vi "Trial 4 A4 copy.vi"() -> ()   [LabVIEW 2022 SP3]
uses:
  Documents/Control 1 Trial 3.ctl
panel:
  out "Time remaining":dbl
  in  "Start":bool
  in  "Stop":bool
  in  "Washing Mode Menu":T1(ring)
  out "Washing Stage":string
  out "Washing Mode":string
  in  "On/Off":bool
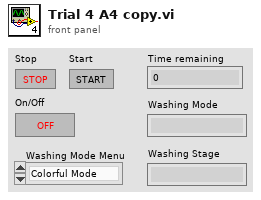
[diagram p1: front panel]
types:
  T1 = enum16{"Colorful Mode", "Intensive Mode", "Quick Wash"}
  T2 = typedef "Control 1 Trial 3.ctl" = enum16{"Off", "On", "Start Washing", "Pre-rinse", "Main Washing", "Final Spin", "Done Washing"}
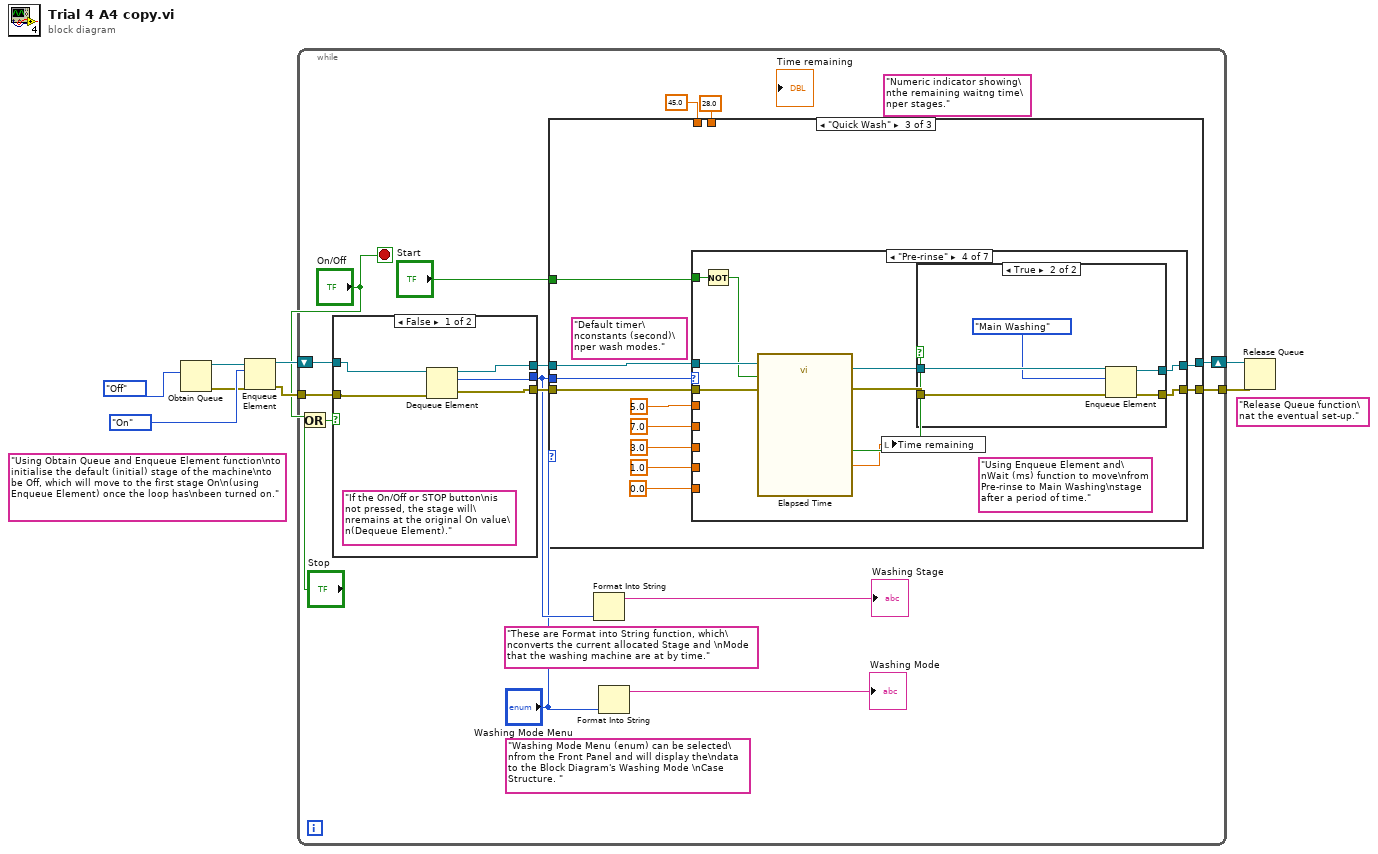
[diagram p0: block diagram]
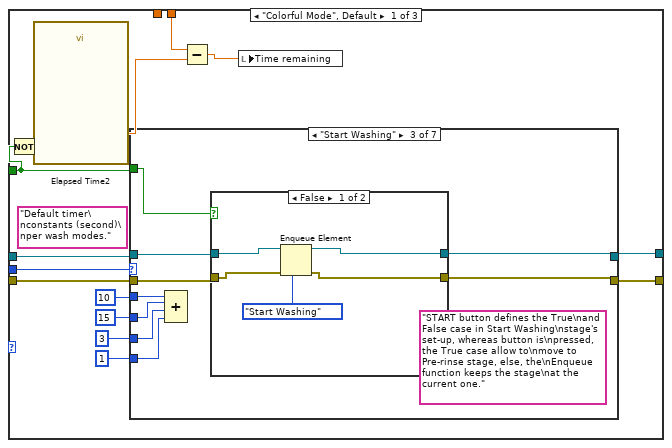
[diagram p2: hidden frame]
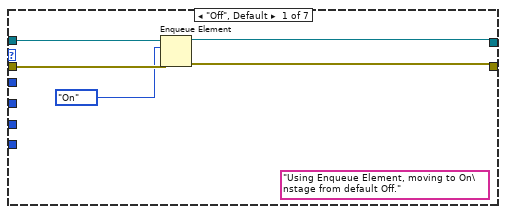
[diagram p3: hidden frame]
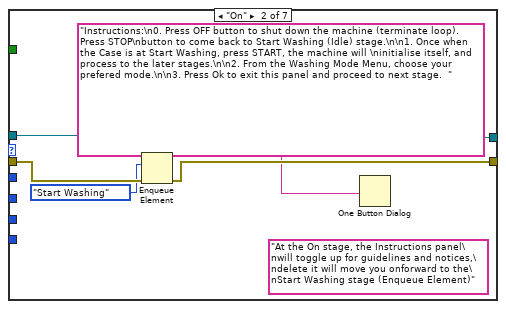
[diagram p4: hidden frame]
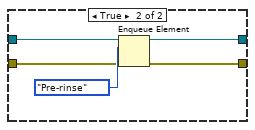
[diagram p5: hidden frame]
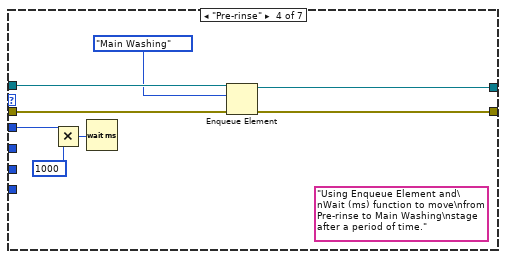
[diagram p6: hidden frame]
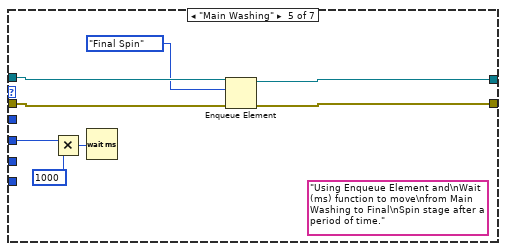
[diagram p7: hidden frame]
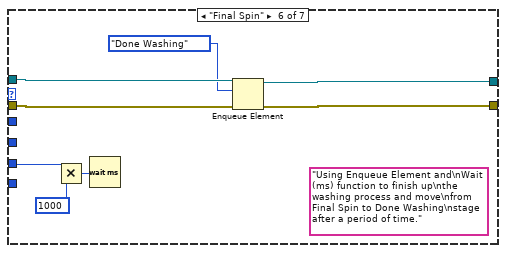
[diagram p8: hidden frame]
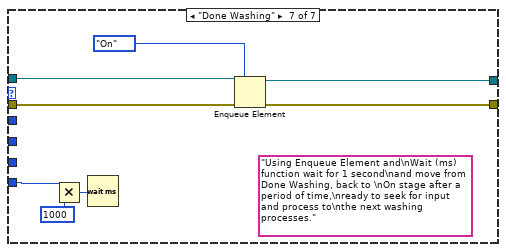
[diagram p9: hidden frame]
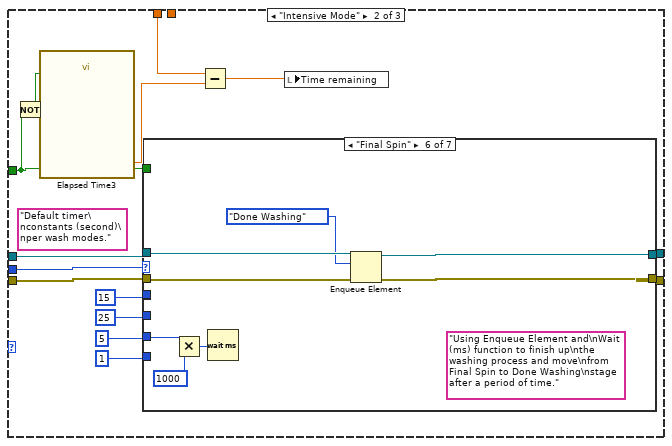
[diagram p10: hidden frame]
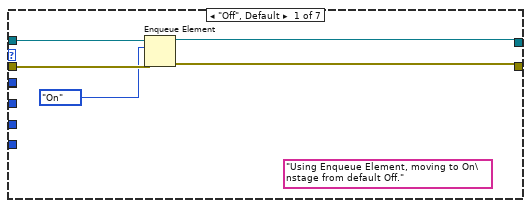
[diagram p11: hidden frame]
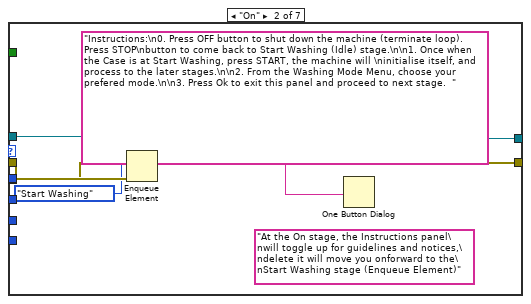
[diagram p12: hidden frame]
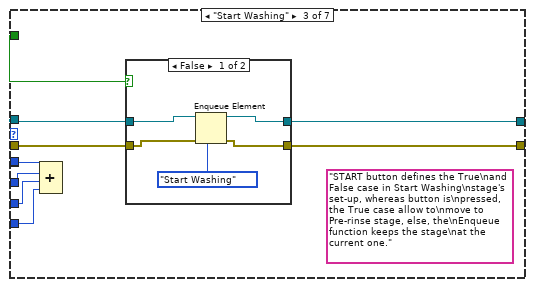
[diagram p13: hidden frame]
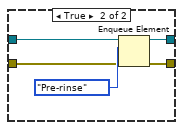
[diagram p14: hidden frame]
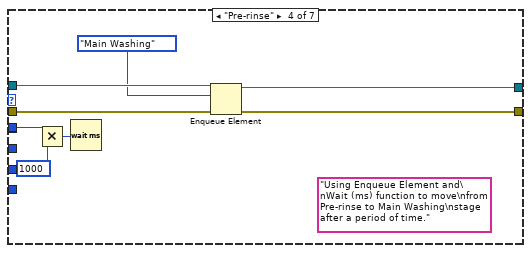
[diagram p15: hidden frame]
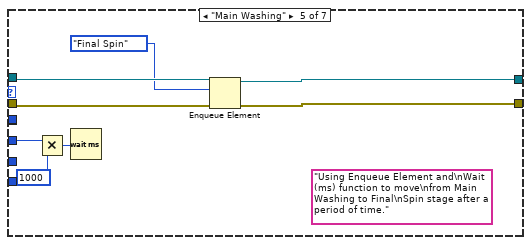
[diagram p16: hidden frame]
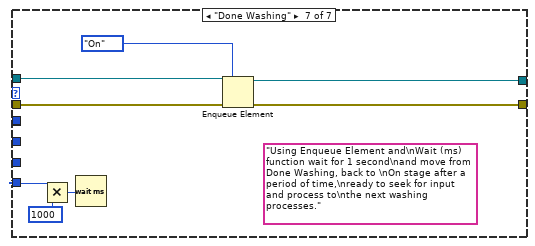
[diagram p17: hidden frame]
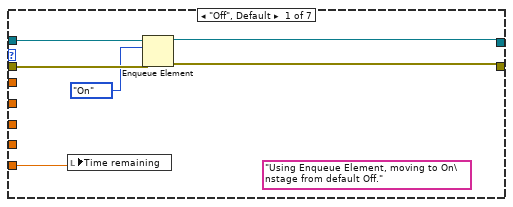
[diagram p18: hidden frame]
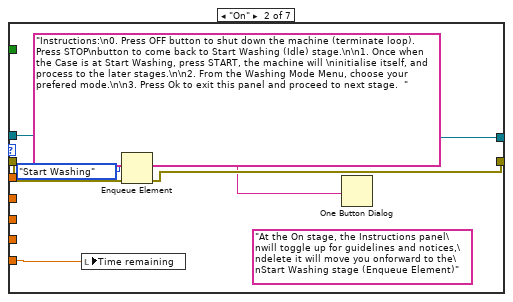
[diagram p19: hidden frame]
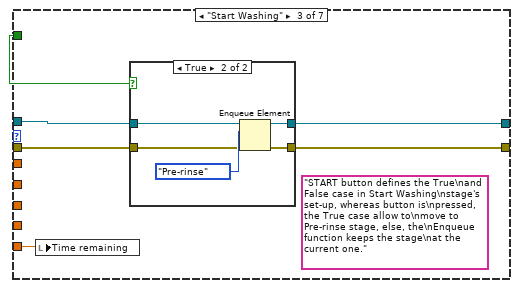
[diagram p20: hidden frame]
diagram:
  (unwired) "Release Queue function\nat the eventual set-up."
  (unwired) "Using Obtain Queue and Enqueue Element function\nto initialise the default (initial) stage of the machine\nto be Off, which will move to the first stage On\n(using Enqueue Element) once the loop has\nbeen turned on."
  n1 = Obtain Queue(element data type=Control_1_Trial_3."Off") -> (queue out=w8:refnum<queue>, error out=w2:errorcluster)  [unwired: 4 in, 1 out]
  n2 = Enqueue Element(queue=w8, element=Control_1_Trial_3."On", error in (no error)=w2) -> (queue out=w7:refnum<queue>, error out=w1:errorcluster)  [unwired: 1 in, 1 out]
  n3 = while {
    shift-right: [w18] -> w5
    shift-left: w7 -> [w23]
    tunnel: w1 -> [w24]
    tunnel: [w17] -> w6
    stop <- "On/Off" stop-if-true
    (unwired) "Numeric indicator showing\nthe remaining waitng time\nper stages."
    (unwired) "Washing Mode Menu (enum) can be selected\nfrom the Front Panel and will display the\ndata to the Block Diagram's Washing Mode \nCase Structure. "
    (unwired) "These are Format into String function, which\nconverts the current allocated Stage and \nMode that the washing machine are at by time."
    n4 = Or(x="On/Off", y="Stop") -> (x .or. y?=w16:bool)
    n5 = case shown="False" w16 {
      tunnel: w24 -> [w291 w296]
      tunnel: w23 -> [w292 w297]
      tunnel: [w288 w294] -> w21
      tunnel: [w289 w295] -> w20
      tunnel: [w290 Control_1_Trial_3."Off"] -> w15
      frame False {
        (unwired) "If the On/Off or STOP button\nis not pressed, the stage will\nremains at the original On value\n(Dequeue Element)."
        n6 = Dequeue Element(queue=w292, error in (no error)=w291) -> (queue out=w288:refnum<queue>, element=w290:T2, error out=w289:errorcluster)  [unwired: 1 in, 1 out]
      }
      frame True {
        (unwired) "Else if the On/Off or STOP button\nis  pressed, the stage will then\nmove to Off value (Flush Queue)."
        n7 = Flush Queue(queue=w297, error in (no error)=w296) -> (queue out=w294:refnum<queue>, error out=w295:errorcluster)  [unwired: 1 out]
      }
    }
    n8 = case shown="\"Quick Wash\"" "Washing Mode Menu" {
      tunnel: w21 -> [w38 w114 w187]
      tunnel: [w35 w113 w185] -> w18
      tunnel: w20 -> [w37 w112 w186]
      tunnel: [w34 w111 w179] -> w17
      tunnel: w15 -> [w36 w110 w180]
      tunnel: "Start" -> [w29 w104 w178]
      tunnel: 45.0 -> [_ w102 _]
      tunnel: 28.0 -> [w26 _ _]
      frame "Colorful Mode", Default {
        (unwired) "Default timer\nconstants (second)\nper wash modes."
        n9 = Not(x=w29) -> (.not. x?=w28:bool)
        n10 = call "Elapsed Time2"("Reset"=w28) -> ("Elapsed Time (s)"=w27:dbl)  [unwired: 11 in, 7 out]
        n11 = case shown="\"Start Washing\"" w36 {
          tunnel: w38 -> [w43 w49 w58 w76 w84 w92 w98]
          tunnel: [w40 w48 w56 w74 w82 w90 w100] -> w35
          tunnel: w37 -> [w42 w47 w57 w75 w83 w91 w97]
          tunnel: [w41 w46 w55 w73 w81 w89 w99] -> w34
          tunnel: 15 -> [_ _ w52 _ w77 _ _]
          tunnel: 3 -> [_ _ w51 _ _ w85 _]
          tunnel: 1 -> [_ _ w50 _ _ _ w93]
          tunnel: 10 -> [_ _ w53 w71 _ _ _]
          tunnel: w29 -> [_ _ w54 _ _ _ _]
          frame "Off", Default {
            (unwired) "Using Enqueue Element, moving to On\nstage from default Off."
            n12 = Enqueue Element(queue=w43, element=Control_1_Trial_3."On", error in (no error)=w42) -> (queue out=w40:refnum<queue>, error out=w41:errorcluster)  [unwired: 1 in, 1 out]
          }
          frame "On" {
            (unwired) "At the On stage, the Instructions panel\nwill toggle up for guidelines and notices,\ndelete it will move you onforward to the\nStart Washing stage (Enqueue Element)"
            n13 = Enqueue Element(queue=w49, element=Control_1_Trial_3."Start Washing", error in (no error)=w47) -> (queue out=w48:refnum<queue>, error out=w46:errorcluster)  [unwired: 1 in, 1 out]
            n14 = One Button Dialog(message="Instructions:\n0. Press OFF button to shut down the machine (terminate loop). Press STOP\nbutton to come back to Start Washing (Idle) stage.\n\n1. Once when the Case is at Start Washing, press START, the machine will \ninitialise itself, and process to the later stages.\n\n2. From the Washing Mode Menu, choose your prefered mode.\n\n3. Press Ok to exit this panel and proceed to next stage.  ") -> ()  [unwired: 1 in, 1 out]
          }
          frame "Start Washing" {
            (unwired) "START button defines the True\nand False case in Start Washing\nstage's set-up, whereas button is\npressed, the True case allow to\nmove to Pre-rinse stage, else, the\nEnqueue function keeps the stage\nat the current one."
            n15 = Compound Arithmetic op=unknown(w53, w52, w51, w50) -> ()  [unwired: 1 out]
            n16 = case shown="False" w54 {
              tunnel: w58 -> [w63 w68]
              tunnel: w57 -> [w62 w66]
              tunnel: [w60 w65] -> w56
              tunnel: [w61 w64] -> w55
              frame False {
                n17 = Enqueue Element(queue=w63, element=Control_1_Trial_3."Start Washing", error in (no error)=w62) -> (queue out=w60:refnum<queue>, error out=w61:errorcluster)  [unwired: 1 in, 1 out]
              }
              frame True {
                n18 = Enqueue Element(queue=w68, element=Control_1_Trial_3."Pre-rinse", error in (no error)=w66) -> (queue out=w65:refnum<queue>, error out=w64:errorcluster)  [unwired: 1 in, 1 out]
              }
            }
          }
          frame "Pre-rinse" {
            (unwired) "Using Enqueue Element and\nWait (ms) function to move\nfrom Pre-rinse to Main Washing\nstage after a period of time."
            n19 = Multiply(x=w71, y=1000) -> (x*y=w69:i32)
            n20 = Wait (ms)(milliseconds to wait=w69) -> ()  [unwired: 1 out]
            n21 = Enqueue Element(queue=w76, element=Control_1_Trial_3."Main Washing", error in (no error)=w75) -> (queue out=w74:refnum<queue>, error out=w73:errorcluster)  [unwired: 1 in, 1 out]
          }
          frame "Main Washing" {
            (unwired) "Using Enqueue Element and\nWait (ms) function to move\nfrom Main Washing to Final\nSpin stage after a period of time."
            n22 = Multiply(x=w77, y=1000) -> (x*y=w78:i32)
            n23 = Wait (ms)(milliseconds to wait=w78) -> ()  [unwired: 1 out]
            n24 = Enqueue Element(queue=w84, element=Control_1_Trial_3."Final Spin", error in (no error)=w83) -> (queue out=w82:refnum<queue>, error out=w81:errorcluster)  [unwired: 1 in, 1 out]
          }
          frame "Final Spin" {
            (unwired) "Using Enqueue Element and\nWait (ms) function to finish up\nthe washing process and move\nfrom Final Spin to Done Washing\nstage after a period of time."
            n25 = Multiply(x=w85, y=1000) -> (x*y=w86:i32)
            n26 = Wait (ms)(milliseconds to wait=w86) -> ()  [unwired: 1 out]
            n27 = Enqueue Element(queue=w92, element=Control_1_Trial_3."Done Washing", error in (no error)=w91) -> (queue out=w90:refnum<queue>, error out=w89:errorcluster)  [unwired: 1 in, 1 out]
          }
          frame "Done Washing" {
            (unwired) "Using Enqueue Element and\nWait (ms) function wait for 1 second\nand move from Done Washing, back to \nOn stage after a period of time,\nready to seek for input and process to\nthe next washing processes."
            n28 = Multiply(x=w93, y=1000) -> (x*y=w94:i32)
            n29 = Wait (ms)(milliseconds to wait=w94) -> ()  [unwired: 1 out]
            n30 = Enqueue Element(queue=w98, element=Control_1_Trial_3."On", error in (no error)=w97) -> (queue out=w100:refnum<queue>, error out=w99:errorcluster)  [unwired: 1 in, 1 out]
          }
        }
        n31 = Subtract(x=w26, y=w27) -> (x-y=w25:dbl)
        n32 = local write "Time remaining"(w25) -> ()
      }
      frame "Intensive Mode" {
        (unwired) "Default timer\nconstants (second)\nper wash modes."
        w106 = 15
        n33 = Not(x=w104) -> (.not. x?=w105:bool)
        n34 = call "Elapsed Time3"("Reset"=w105) -> ("Elapsed Time (s)"=w103:dbl)  [unwired: 11 in, 7 out]
        n35 = case shown="\"Final Spin\"" w110 {
          tunnel: w114 -> [w119 w125 w132 w152 w160 w168 w174]
          tunnel: [w116 w124 w134 w150 w158 w166 w176] -> w113
          tunnel: w112 -> [w118 w123 w131 w151 w159 w167 w173]
          tunnel: [w117 w122 w133 w149 w157 w165 w175] -> w111
          tunnel: w106 -> [_ _ w129 _ _ _ _]
          tunnel: 25 -> [_ _ w128 _ w153 _ _]
          tunnel: 5 -> [_ _ w127 _ _ w161 _]
          tunnel: 1 -> [_ _ w126 _ _ _ w169]
          tunnel: w106 -> [_ _ _ w147 _ _ _]
          tunnel: w104 -> [_ _ w130 _ _ _ _]
          frame "Off", Default {
            (unwired) "Using Enqueue Element, moving to On\nstage from default Off."
            n36 = Enqueue Element(queue=w119, element=Control_1_Trial_3."On", error in (no error)=w118) -> (queue out=w116:refnum<queue>, error out=w117:errorcluster)  [unwired: 1 in, 1 out]
          }
          frame "On" {
            (unwired) "At the On stage, the Instructions panel\nwill toggle up for guidelines and notices,\ndelete it will move you onforward to the\nStart Washing stage (Enqueue Element)"
            n37 = Enqueue Element(queue=w125, element=Control_1_Trial_3."Start Washing", error in (no error)=w123) -> (queue out=w124:refnum<queue>, error out=w122:errorcluster)  [unwired: 1 in, 1 out]
            n38 = One Button Dialog(message="Instructions:\n0. Press OFF button to shut down the machine (terminate loop). Press STOP\nbutton to come back to Start Washing (Idle) stage.\n\n1. Once when the Case is at Start Washing, press START, the machine will \ninitialise itself, and process to the later stages.\n\n2. From the Washing Mode Menu, choose your prefered mode.\n\n3. Press Ok to exit this panel and proceed to next stage.  ") -> ()  [unwired: 1 in, 1 out]
          }
          frame "Start Washing" {
            (unwired) "START button defines the True\nand False case in Start Washing\nstage's set-up, whereas button is\npressed, the True case allow to\nmove to Pre-rinse stage, else, the\nEnqueue function keeps the stage\nat the current one."
            n39 = Compound Arithmetic op=unknown(w129, w128, w127, w126) -> ()  [unwired: 1 out]
            n40 = case shown="False" w130 {
              tunnel: w132 -> [w139 w144]
              tunnel: w131 -> [w138 w142]
              tunnel: [w136 w141] -> w134
              tunnel: [w137 w140] -> w133
              frame False {
                n41 = Enqueue Element(queue=w139, element=Control_1_Trial_3."Start Washing", error in (no error)=w138) -> (queue out=w136:refnum<queue>, error out=w137:errorcluster)  [unwired: 1 in, 1 out]
              }
              frame True {
                n42 = Enqueue Element(queue=w144, element=Control_1_Trial_3."Pre-rinse", error in (no error)=w142) -> (queue out=w141:refnum<queue>, error out=w140:errorcluster)  [unwired: 1 in, 1 out]
              }
            }
          }
          frame "Pre-rinse" {
            (unwired) "Using Enqueue Element and\nWait (ms) function to move\nfrom Pre-rinse to Main Washing\nstage after a period of time."
            n43 = Multiply(x=w147, y=1000) -> (x*y=w145:i32)
            n44 = Wait (ms)(milliseconds to wait=w145) -> ()  [unwired: 1 out]
            n45 = Enqueue Element(queue=w152, element=Control_1_Trial_3."Main Washing", error in (no error)=w151) -> (queue out=w150:refnum<queue>, error out=w149:errorcluster)  [unwired: 1 in, 1 out]
          }
          frame "Main Washing" {
            (unwired) "Using Enqueue Element and\nWait (ms) function to move\nfrom Main Washing to Final\nSpin stage after a period of time."
            n46 = Multiply(x=w153, y=1000) -> (x*y=w154:i32)
            n47 = Wait (ms)(milliseconds to wait=w154) -> ()  [unwired: 1 out]
            n48 = Enqueue Element(queue=w160, element=Control_1_Trial_3."Final Spin", error in (no error)=w159) -> (queue out=w158:refnum<queue>, error out=w157:errorcluster)  [unwired: 1 in, 1 out]
          }
          frame "Final Spin" {
            (unwired) "Using Enqueue Element and\nWait (ms) function to finish up\nthe washing process and move\nfrom Final Spin to Done Washing\nstage after a period of time."
            n49 = Multiply(x=w161, y=1000) -> (x*y=w162:i32)
            n50 = Wait (ms)(milliseconds to wait=w162) -> ()  [unwired: 1 out]
            n51 = Enqueue Element(queue=w168, element=Control_1_Trial_3."Done Washing", error in (no error)=w167) -> (queue out=w166:refnum<queue>, error out=w165:errorcluster)  [unwired: 1 in, 1 out]
          }
          frame "Done Washing" {
            (unwired) "Using Enqueue Element and\nWait (ms) function wait for 1 second\nand move from Done Washing, back to \nOn stage after a period of time,\nready to seek for input and process to\nthe next washing processes."
            n52 = Multiply(x=w169, y=1000) -> (x*y=w170:i32)
            n53 = Wait (ms)(milliseconds to wait=w170) -> ()  [unwired: 1 out]
            n54 = Enqueue Element(queue=w174, element=Control_1_Trial_3."On", error in (no error)=w173) -> (queue out=w176:refnum<queue>, error out=w175:errorcluster)  [unwired: 1 in, 1 out]
          }
        }
        n55 = Subtract(x=w102, y=w103) -> (x-y=w101:dbl)
        n56 = local write "Time remaining"(w101) -> ()
      }
      frame "Quick Wash" {
        (unwired) "Default timer\nconstants (second)\nper wash modes."
        n57 = case shown="\"Pre-rinse\"" w180 {
          tunnel: w187 -> [w193 w200 w206 w224 w242 w259 w275]
          tunnel: [w191 w199 w204 w223 w240 w257 w277] -> w185
          tunnel: w186 -> [w190 w198 w205 w219 w241 w258 w274]
          tunnel: [w192 w197 w203 w222 w239 w256 w276] -> w179
          tunnel: 7.0 -> [_ _ _ _ w237 _ _]
          tunnel: 3.0 -> [_ _ _ _ _ w255 _]
          tunnel: 1.0 -> [_ _ _ _ _ _ w272]
          tunnel: 5.0 -> [_ _ _ _ _ _ _]
          tunnel: w178 -> [_ _ w202 w221 _ _ _]
          tunnel: 0.0 -> [w188 w194 w201 _ _ _ _]
          frame "Off", Default {
            (unwired) "Using Enqueue Element, moving to On\nstage from default Off."
            n58 = local write "Time remaining"(w188) -> ()
            n59 = Enqueue Element(queue=w193, element=Control_1_Trial_3."On", error in (no error)=w190) -> (queue out=w191:refnum<queue>, error out=w192:errorcluster)  [unwired: 1 in, 1 out]
          }
          frame "On" {
            (unwired) "At the On stage, the Instructions panel\nwill toggle up for guidelines and notices,\ndelete it will move you onforward to the\nStart Washing stage (Enqueue Element)"
            n60 = local write "Time remaining"(w194) -> ()
            n61 = Enqueue Element(queue=w200, element=Control_1_Trial_3."Start Washing", error in (no error)=w198) -> (queue out=w199:refnum<queue>, error out=w197:errorcluster)  [unwired: 1 in, 1 out]
            n62 = One Button Dialog(message="Instructions:\n0. Press OFF button to shut down the machine (terminate loop). Press STOP\nbutton to come back to Start Washing (Idle) stage.\n\n1. Once when the Case is at Start Washing, press START, the machine will \ninitialise itself, and process to the later stages.\n\n2. From the Washing Mode Menu, choose your prefered mode.\n\n3. Press Ok to exit this panel and proceed to next stage.  ") -> ()  [unwired: 1 in, 1 out]
          }
          frame "Start Washing" {
            (unwired) "START button defines the True\nand False case in Start Washing\nstage's set-up, whereas button is\npressed, the True case allow to\nmove to Pre-rinse stage, else, the\nEnqueue function keeps the stage\nat the current one."
            n63 = local write "Time remaining"(w201) -> ()
            n64 = case shown="True" w202 {
              tunnel: w206 -> [w211 w216]
              tunnel: w205 -> [w210 w214]
              tunnel: [w208 w213] -> w204
              tunnel: [w209 w212] -> w203
              frame False {
                n65 = Enqueue Element(queue=w211, element=Control_1_Trial_3."Start Washing", error in (no error)=w210) -> (queue out=w208:refnum<queue>, error out=w209:errorcluster)  [unwired: 1 in, 1 out]
              }
              frame True {
                n66 = Enqueue Element(queue=w216, element=Control_1_Trial_3."Pre-rinse", error in (no error)=w214) -> (queue out=w213:refnum<queue>, error out=w212:errorcluster)  [unwired: 1 in, 1 out]
              }
            }
          }
          frame "Pre-rinse" {
            (unwired) "Using Enqueue Element and\nWait (ms) function to move\nfrom Pre-rinse to Main Washing\nstage after a period of time."
            n67 = Not(x=w221) -> (.not. x?=w220:bool)
            n68 = call "Elapsed Time"("Reset"=w220) -> ("Elapsed Time (s)"=w217:dbl, "Time has Elapsed"=w218:bool)  [unwired: 11 in, 6 out]
            n69 = local write "Time remaining"(w217) -> ()
            n70 = case shown="True" w218 {
              tunnel: w224 -> [w229 w234]
              tunnel: w219 -> [w227 w233]
              tunnel: [w228 w232] -> w223
              tunnel: [w226 w231] -> w222
              frame False {
                n71 = Enqueue Element(queue=w229, element=Control_1_Trial_3."Pre-rinse", error in (no error)=w227) -> (queue out=w228:refnum<queue>, error out=w226:errorcluster)  [unwired: 1 in, 1 out]
              }
              frame True {
                n72 = Enqueue Element(queue=w234, element=Control_1_Trial_3."Main Washing", error in (no error)=w233) -> (queue out=w232:refnum<queue>, error out=w231:errorcluster)  [unwired: 1 in, 1 out]
              }
            }
          }
          frame "Main Washing" {
            (unwired) "Using Enqueue Element and\nWait (ms) function to move\nfrom Main Washing to Final\nSpin stage after a period of time."
            n73 = call "Elapsed Time4"() -> ("Elapsed Time (s)"=w236:dbl, "Time has Elapsed"=w238:bool)  [unwired: 12 in, 6 out]
            n74 = Subtract(x=w237, y=w236) -> (x-y=w235:dbl)
            n75 = case shown="False" w238 {
              tunnel: w242 -> [w247 w252]
              tunnel: w241 -> [w245 w251]
              tunnel: [w246 w250] -> w240
              tunnel: [w244 w249] -> w239
              frame False {
                n76 = Enqueue Element(queue=w247, element=Control_1_Trial_3."Main Washing", error in (no error)=w245) -> (queue out=w246:refnum<queue>, error out=w244:errorcluster)  [unwired: 1 in, 1 out]
              }
              frame True {
                n77 = Enqueue Element(queue=w252, element=Control_1_Trial_3."Final Spin", error in (no error)=w251) -> (queue out=w250:refnum<queue>, error out=w249:errorcluster)  [unwired: 1 in, 1 out]
              }
            }
            n78 = local write "Time remaining"(w235) -> ()
          }
          frame "Final Spin" {
            (unwired) "Using Enqueue Element and\nWait (ms) function to finish up\nthe washing process and move\nfrom Final Spin to Done Washing\nstage after a period of time."
            n79 = call "Elapsed Time5"() -> ("Elapsed Time (s)"=w254:dbl, "Time has Elapsed"=w253:bool)  [unwired: 12 in, 6 out]
            n80 = Subtract(x=w255, y=w254) -> ()  [unwired: 1 out]
            n81 = case shown="False" w253 {
              tunnel: w259 -> [w264 w269]
              tunnel: w258 -> [w262 w268]
              tunnel: [w263 w267] -> w257
              tunnel: [w261 w266] -> w256
              frame False {
                n82 = Enqueue Element(queue=w264, element=Control_1_Trial_3."Final Spin", error in (no error)=w262) -> (queue out=w263:refnum<queue>, error out=w261:errorcluster)  [unwired: 1 in, 1 out]
              }
              frame True {
                n83 = Enqueue Element(queue=w269, element=Control_1_Trial_3."Done Washing", error in (no error)=w268) -> (queue out=w267:refnum<queue>, error out=w266:errorcluster)  [unwired: 1 in, 1 out]
              }
            }
          }
          frame "Done Washing" {
            (unwired) "Using Enqueue Element and\nWait (ms) function wait for 1 second\nand move from Done Washing, back to \nOn stage after a period of time,\nready to seek for input and process to\nthe next washing processes."
            n84 = call "Elapsed Time6"() -> ("Elapsed Time (s)"=w273:dbl, "Time has Elapsed"=w270:bool)  [unwired: 12 in, 6 out]
            n85 = Subtract(x=w272, y=w273) -> (x-y=w271:dbl)
            n86 = local write "Time remaining"(w271) -> ()
            n87 = case shown="False" w270 {
              tunnel: [w281 w287] -> w277
              tunnel: [w279 w286] -> w276
              tunnel: w275 -> [w282 w285]
              tunnel: w274 -> [w280 w284]
              frame False {
                n88 = Enqueue Element(queue=w282, element=Control_1_Trial_3."Done Washing", error in (no error)=w280) -> (queue out=w281:refnum<queue>, error out=w279:errorcluster)  [unwired: 1 in, 1 out]
              }
              frame True {
                n89 = Enqueue Element(queue=w285, element=Control_1_Trial_3."On", error in (no error)=w284) -> (queue out=w287:refnum<queue>, error out=w286:errorcluster)  [unwired: 1 in, 1 out]
              }
            }
          }
        }
      }
    }
    n90 = Format Into String(w15) -> (resulting string=→"Washing Stage":string)  [unwired: 3 in, 1 out]
    n91 = Format Into String("Washing Mode Menu") -> (resulting string=→"Washing Mode":string)  [unwired: 3 in, 1 out]
  }
  n92 = Release Queue(queue=w5, error in (no error)=w6) -> ()  [unwired: 1 in, 3 out]
